vi "Network Steam Close.vi"(8 "error in (no error)":errorcluster, 11 "Model in":refnum<class "Model.lvclass">) -> (0 "error out":errorcluster, 3 "Model out":refnum<class "Model.lvclass">)   [LabVIEW 2021, in "Model.lvlib" / "Model.lvclass"]
uses:
  Model.lvclass
  Model.lvclass/Model.ctl
  <userlib>/John_Lib/Network_Streams_Connection/NetworkConnection.lvclass
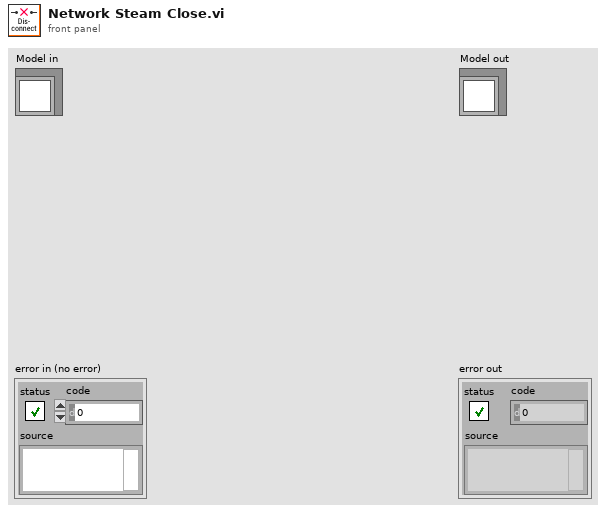
[diagram p1: front panel]
types:
  T1 = typedef "Model.lvlib/Model.lvclass/DVR.ctl" = cluster{"JKI_Network_Streams":refnum<class "NetworkConnection.lvclass">}
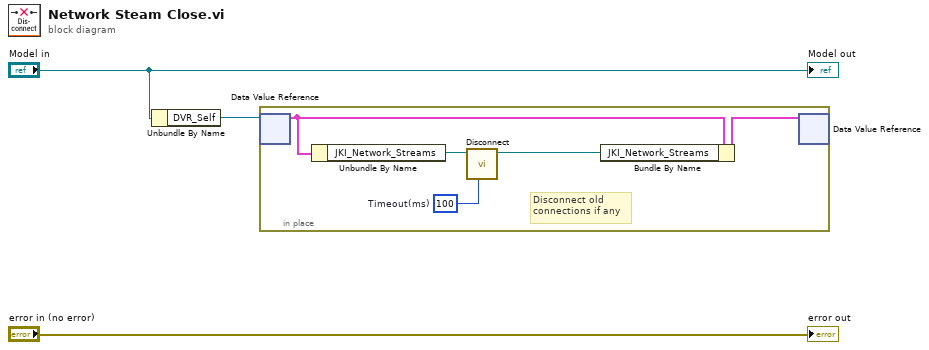
[diagram p0: block diagram]
diagram:
  n1 = Unbundle By Name("Model in") -> ("DVR_Self"=w1:refnum<data-value>)
  n2 = in-place {
    w8 = 100  # Timeout(ms)
    # "Disconnect old\nconnections if any"
    n3 = in-place-dvr #1(w1) -> (w7:T1)  [unwired: 1 out]
    n4 = Unbundle By Name(w7) -> ("JKI_Network_Streams"=w6:refnum<class "NetworkConnection.lvclass">)
    n5 = call <userlib>:"Disconnect.vi"("Timeout ms (1000)"=w8, "NetworkConnection in"=w6) -> ("NetworkConnection out"=w4:refnum<class "NetworkConnection.lvclass">)  [unwired: 8 in, 1 out]
    n6 = Bundle By Name(cluster=w7, "JKI_Network_Streams"=w4) -> (w5:T1)
    n7 = in-place-dvr #1(w5) -> ()  [unwired: 2 out]
  }
  "error out" <- "error in (no error)"
  "Model out" <- "Model in"
